vi "message.vi"() -> ()   [LabVIEW 2010]
panel:
  in  "Galil.IGalil":refnum<k7>
  out "OFFLINE error":errorcluster
  in  "stop_vi":bool
  out "message":string
  out "Library Version:":string
  out "error out":errorcluster
  out "Connected To:":string
  in  "Connection String:":string
  # "This vi Shows how to use the onMessage event of the Galil Communications Library.  \n\nIf Connection String is left blank, the vi will open the connections dialog when run.  If a value is input into Connection String, the vi will attempt to connect to the controller at that address (ex COM1 19200).\n\nThe vi downloads a program to the controller with the programDownload function.  The program sends TIME command as an unsolicited message every 50ms.  The event_message.vi handles the onMessage event and passes the data to the message.vi and displays it in the message string indicator.\n\nThe vi will run until the STOP button is pressed.  The STOP button should be used to stop the VI."
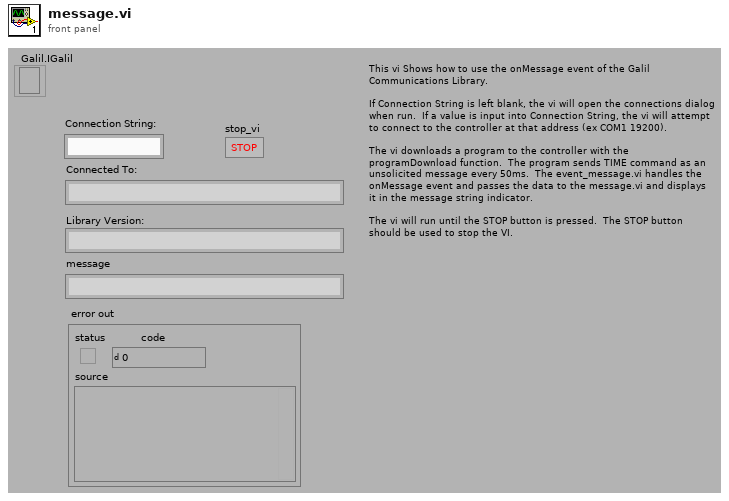
[diagram p1: front panel]
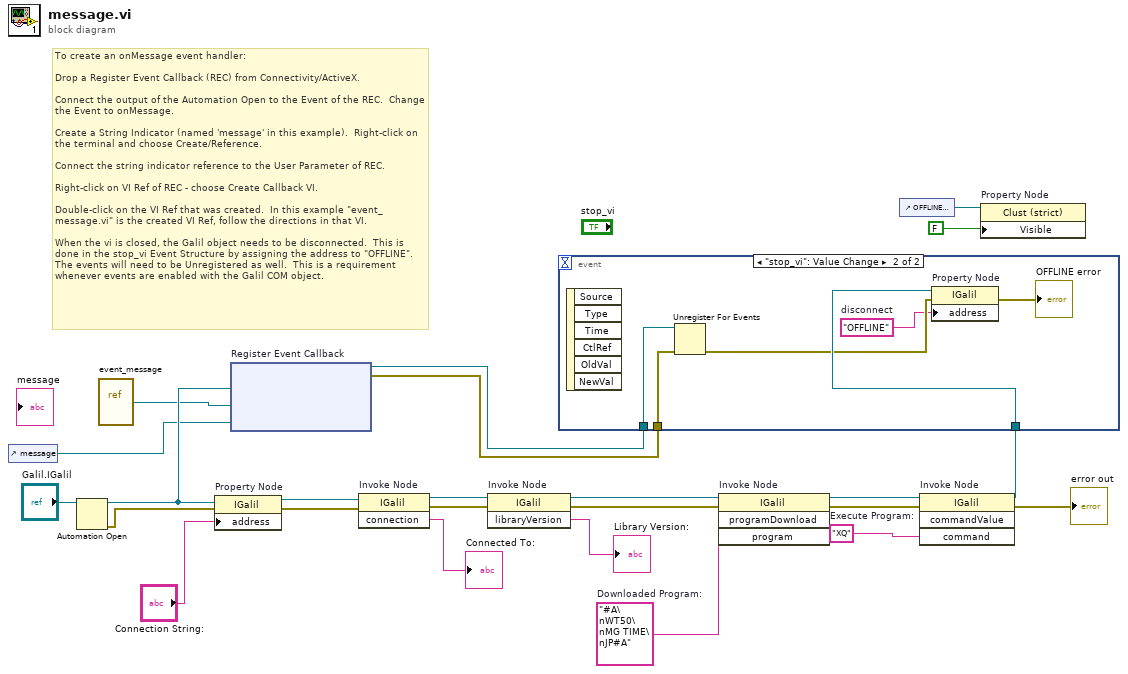
[diagram p0: block diagram]
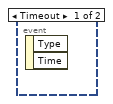
[diagram p2: hidden frame]
diagram:
  w11 = "XQ"  # Execute Program:
  w14 = "#A\nWT50\nMG TIME\nJP#A"  # Downloaded Program:
  # "To create an onMessage event handler:\n\nDrop a Register Event Callback (REC) from Connectivity/ActiveX.  \n\nConnect the output of the Automation Open to the Event of the REC.  Change the Event to onMessage.\n\nCreate a String Indicator (named 'message' in this example).  Right-click on the terminal and choose Create/Reference.\n\nConnect the string indicator reference to the User Parameter of REC.\n\nRight-click on VI Ref of REC - choose Create Callback VI. \n\nDouble-click on the VI Ref that was created.  In this example \"event_message.vi\" is the created VI Ref, follow the directions in that VI.\n\nWhen the vi is closed, the Galil object needs to be disconnected.  This is done in the stop_vi Event Structure by assigning the address to \"OFFLINE\".  The events will need to be Unregistered as well.  This is a requirement whenever events are enabled with the Galil COM object."
  n1 = control-ref of="message"() -> (w9:refnum<vi>)
  n2 = Automation Open(Automation Refnum="Galil.IGalil") -> (Automation Refnum=w10:refnum<k7>, error out=w23:errorcluster)  [unwired: 1 in, 2 out]
  n3 = vi-ref "event_message.vi"() -> ("vi reference"=w8:refnum<vi>)
  n4 = property on="Property Node" class="IGalil"(reference=w10, error in=w23, "address"="Connection String:") -> (reference out=w24:refnum<k7>, error out=w22:errorcluster)
  n5 = node "Register Event Callback"(w10, w8, w9) -> (w5:refnum<k27>, w4:errorcluster)  [unwired: 2 in]
  n6 = invoke on="Invoke Node" class="IGalil" method="connection"(reference=w24, error in=w22) -> (reference out=w17:refnum<k7>, error out=w19:errorcluster, "connection"=→"Connected To:":string)  [unwired: 1 in]
  n7 = invoke on="Invoke Node" class="IGalil" method="libraryVersion"(reference=w17, error in=w19) -> (reference out=w16:refnum<k7>, error out=w15:errorcluster, "libraryVersion"=→"Library Version:":string)  [unwired: 1 in]
  n8 = invoke on="Invoke Node" class="IGalil" method="programDownload"(reference=w16, error in=w15, "program"=w14) -> (reference out=w13:refnum<k7>, error out=w12:errorcluster)  [unwired: 1 in, 2 out]
  n9 = control-ref of="OFFLINE error"() -> (w2:refnum<vi>)
  n10 = invoke on="Invoke Node" class="IGalil" method="commandValue"(reference=w13, error in=w12, "command"=w11) -> (reference out=w7:refnum<k7>, error out=→"error out":errorcluster)  [unwired: 1 in, 2 out]
  n11 = event shown="[1] \"stop_vi\": Value Change" {
    selector: _ -> [_ _]
    dyn-events: _ -> [_ _]
    timeout: _ -> [_ _]
    tunnel: w7 -> [_ w30]
    tunnel: w5 -> [_ w29]
    tunnel: w4 -> [_ w26]
    event Timeout {
      n12 = event-data() -> ()  [unwired: 3 out]
    }
    event "stop_vi": Value Change {
      w25 = "OFFLINE"  # disconnect
      n13 = event-data() -> ()  [unwired: 7 out]
      n14 = Unregister For Events(event registration refnum=w29, error in=w26) -> (error out=w27:errorcluster)
      n15 = property on="Property Node" class="IGalil"(reference=w30, error in=w27, "address"=w25) -> (error out=→"OFFLINE error":errorcluster)  [unwired: 1 out]
    }
  }
  n16 = property on="Property Node" class="Clust (strict)"(reference=w2, "Visible"=FALSE) -> ()  [unwired: 1 in, 2 out]
